vi "Logger Add Log Element.vi"(8 "error in (no error)":errorcluster, 10 "Element":string, 11 "LoggerRef In":T1) -> (0 "error out":errorcluster, 3 "LoggerRef Out":T1)   [LabVIEW 2014]
uses:
  LoggerRef.ctl
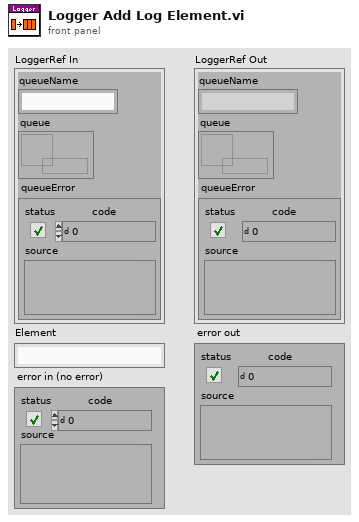
[diagram p1: front panel]
types:
  T1 = typedef "LoggerRef.ctl" = cluster{"queueName":string, "queue":refnum<queue>, "queueError":errorcluster}
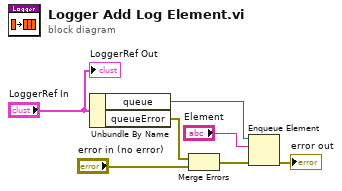
[diagram p0: block diagram]
diagram:
  n1 = Unbundle By Name("LoggerRef In") -> ("queue"=w6:refnum<queue>, "queueError"=w3:errorcluster)
  n2 = Merge Errors(w3, "error in (no error)") -> (w5:errorcluster)
  n3 = Enqueue Element(queue=w6, element="Element", error in (no error)=w5) -> (error out=→"error out":errorcluster)  [unwired: 1 in, 2 out]
  "LoggerRef Out" <- "LoggerRef In"
